vi "File writing training.vi"() -> ()   [LabVIEW 2020]
uses:
  <vilib>/Analysis/Matrix/Numeric/Conversions/Array To Matrix - RA.vi
  <vilib>/Utility/file.llb/Write Delimited Spreadsheet (DBL).vi
  <vilib>/Analysis/Matrix/NI_Matrix.lvlib
panel:
  out "error out":errorcluster
  in  "?":bool
  out "Full filepath":string
  in  "Path":path
  in  "File extension":string
  in  "Filename":string
  in  "Wait time (ms)":dbl
  out "Time":timestamp
  out "?":dbl
  in  "?":bool
  out "Crazyness":dbl(knob) scale=0.0..100000000000000.0
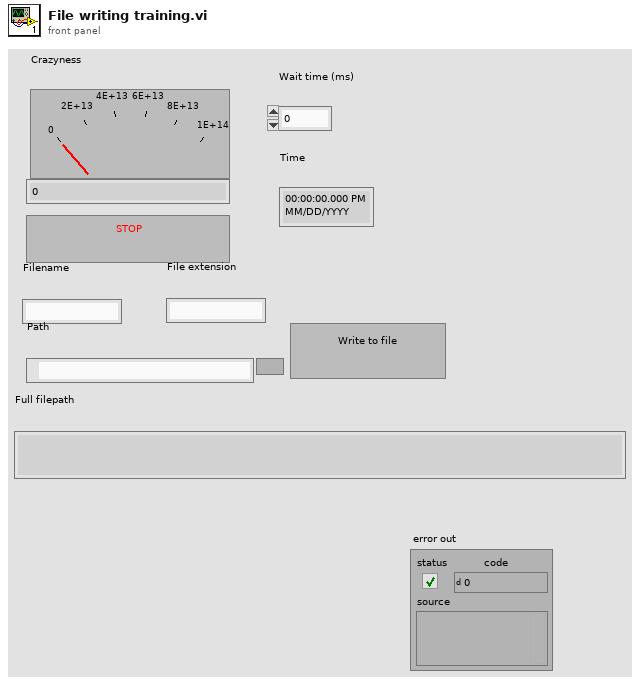
[diagram p1: front panel]
types:
  T1 = typedef "NI_Matrix.lvlib/RealMatrix.ctl" = dbl[][]
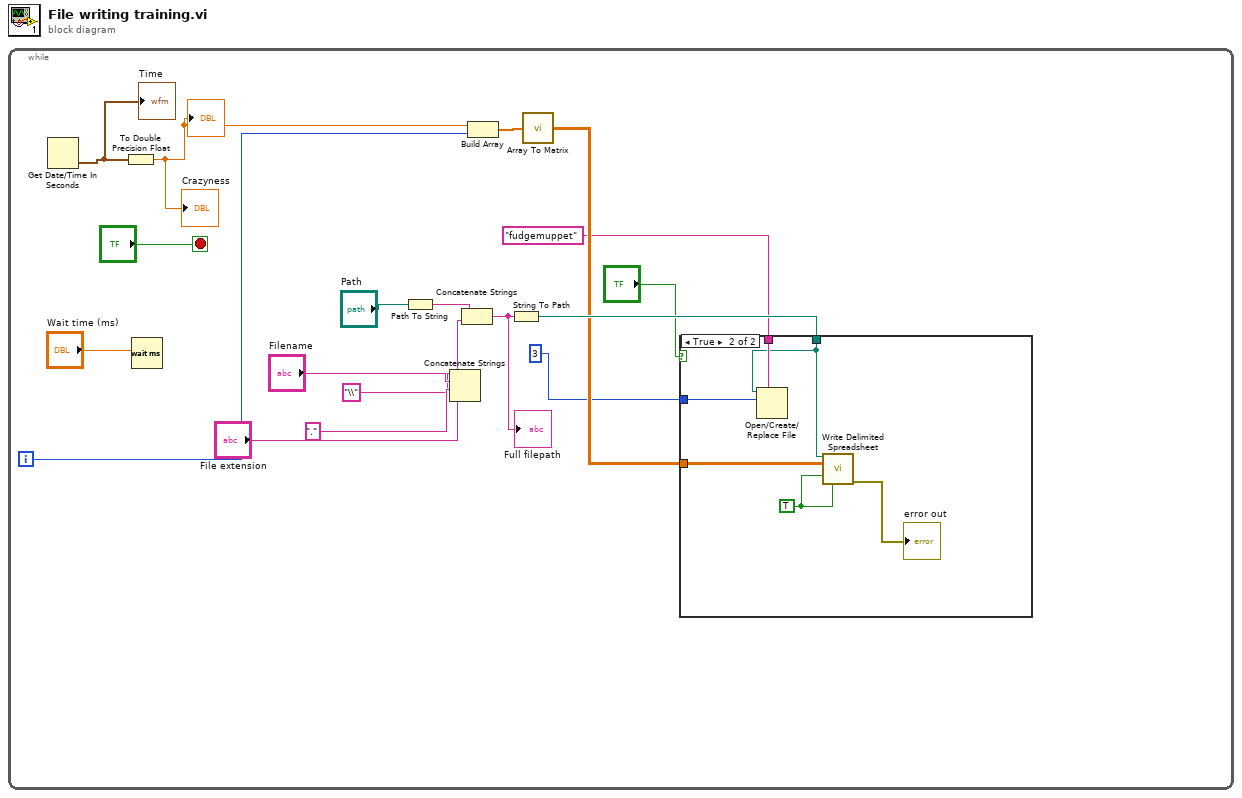
[diagram p0: block diagram]
diagram:
  n1 = while {
    i -> [w7]
    stop <- "?" stop-if-true
    n2 = Get Date/Time In Seconds() -> (seconds since 1Jan1904=w18:timestamp)
    "Time" <- w18
    n3 = To Double Precision Float(number=w18) -> (double precision float=w8:dbl)
    "Crazyness" <- w8
    "?" <- w8
    n4 = Wait (ms)(milliseconds to wait="Wait time (ms)") -> ()  [unwired: 1 out]
    n5 = Path To String(path="Path") -> (string=w15:string)
    n6 = Concatenate Strings("\\", "Filename", ".", "File extension") -> (w14:string)
    n7 = Concatenate Strings(w15, w14) -> (w13:string)
    "Full filepath" <- w13
    n8 = Build Array(w8, w7) -> (w6:dbl[])
    n9 = String To Path(string=w13) -> (path=w5:path)
    n10 = call-poly <vilib>:"Array To Matrix.vi"("Real 1D Array"=w6) -> ("Real Matrix (Column Vector)"=w4:T1)
    n11 = case shown="True" "?" {
      tunnel: w5 -> [_ w22]
      tunnel: w4 -> [_ w25]
      tunnel: "fudgemuppet" -> [_ w24]
      tunnel: 3 -> [_ w23]
      frame False {
      }
      frame True {
        w20 = TRUE
        n12 = Open/Create/Replace File(file path (use dialog)=w22, prompt=w24, operation (0:open)=w23) -> ()  [unwired: 3 in, 3 out]
        n13 = call-poly <vilib>:"Write Delimited Spreadsheet.vi"("file path (dialog if empty)"=w22, "2D data"=w25, "append to file? (new file:F)"=w20, "transpose? (no:F)"=w20) -> ("error out"=→"error out":errorcluster)  [unwired: 10 in, 1 out]
      }
    }
  }
